vi "lockin - Set REF phase equals zero.vi"(8 "error in (no error)":errorcluster, 11 "Lockin":refnum<class "Instrument.Lockin.lvclass">) -> (0 "error out":errorcluster, 3 "Lockin out":refnum<class "Instrument.Lockin.lvclass">)   [LabVIEW 2016, in "Instrument.Lockin.lvclass"]
uses:
  Instrument.Lockin.lvclass
  Instrument.Lockin.lvclass/Instrument.Lockin.ctl
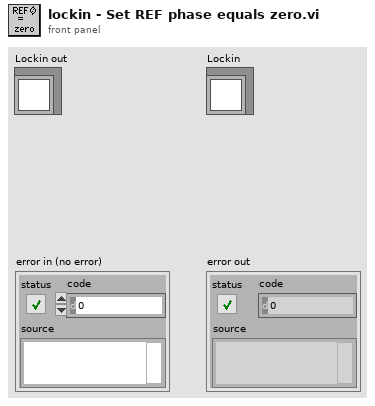
[diagram p1: front panel]
types:
  T1 = typedef "Instrument.Lockin.lvclass/REF_phi-array.ctl" = dbl[]
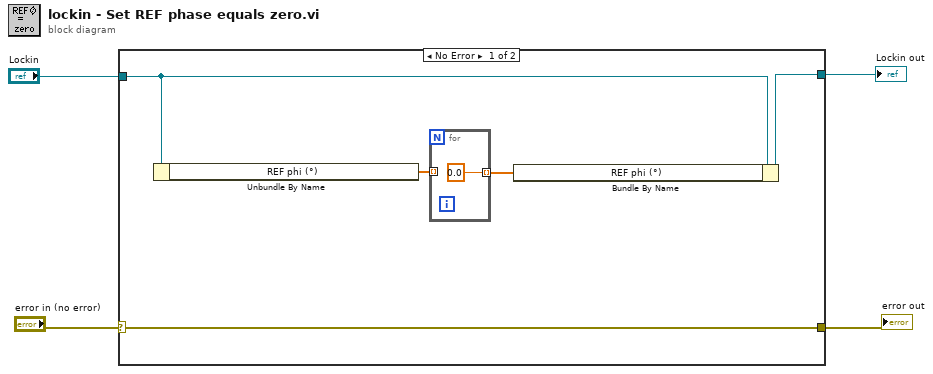
[diagram p0: block diagram]
diagram:
  n1 = case shown="No Error" "error in (no error)" {
    selector: "error in (no error)" -> [w5 w12]
    tunnel: "Lockin" -> [w9 w11]
    tunnel: [w8 w11] -> w3
    tunnel: [w5 w12] -> w1
    frame No Error {
      n2 = Unbundle By Name(w9) -> ("REF phi (°)"=w7:T1)
      n3 = for {
        tunnel: [0.0] -> w6 mode=indexing
        tunnel: w7 -> [_] mode=indexing
      }
      n4 = Bundle By Name(cluster=w9, "REF phi (°)"=w6) -> (w8:refnum<class "Instrument.Lockin.lvclass">)
    }
    frame Error {
    }
  }
  "Lockin out" <- w3
  "error out" <- w1
